vi "StrSplit.vi"(2 "token":string, 3 "str in":string) -> (0 "len":i32, 1 "str out":string[](array[string]))   [LabVIEW 2012]
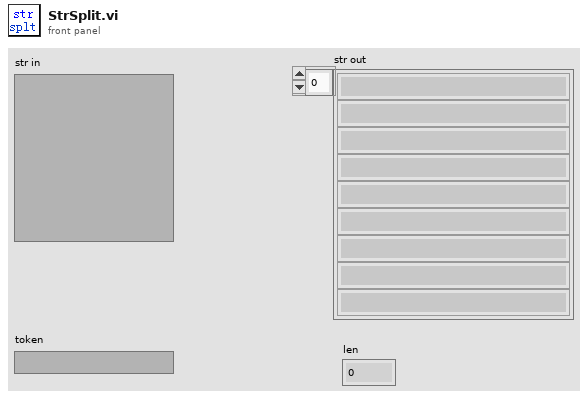
[diagram p1: front panel]
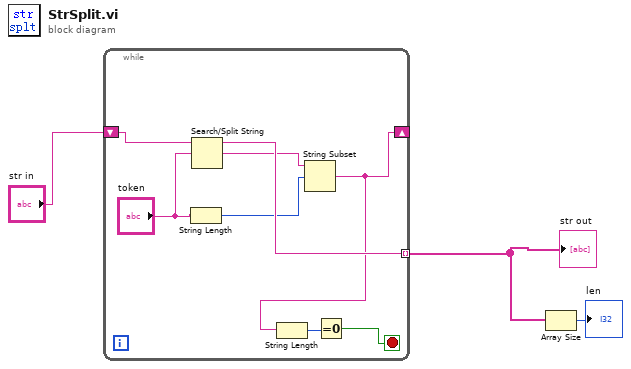
[diagram p0: block diagram]
diagram:
  n1 = while {
    shift-right: [w6] -> _
    shift-left: "str in" -> [w11]
    tunnel: [w10] -> w1 mode=indexing
    stop <- w4 stop-if-true
    n2 = String Length(string="token") -> (length=w7:i32)
    n3 = Search/Split String(string=w11, search string/char (-)="token") -> (substring before match=w10:string, match + rest of string=w8:string)  [unwired: 1 in, 1 out]
    n4 = String Subset(string=w8, offset (0)=w7) -> (substring=w6:string)  [unwired: 1 in]
    n5 = String Length(string=w6) -> (length=w5:i32)
    n6 = Equal To 0?(x=w5) -> (x = 0?=w4:bool)
  }
  "str out" <- w1
  n7 = Array Size(array=w1) -> (size(s)=→"len":i32)
